vi "Task Killer (pid).vi"(4 "Error In":errorcluster, 6 "Force Kill?":bool, 7 "PID":i32) -> (0 "Error Out":errorcluster)   [LabVIEW 2014, in "Managing Executables.lvlib"]
uses:
  Managing Executables.lvlib
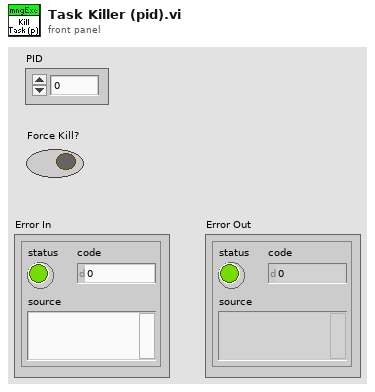
[diagram p1: front panel]
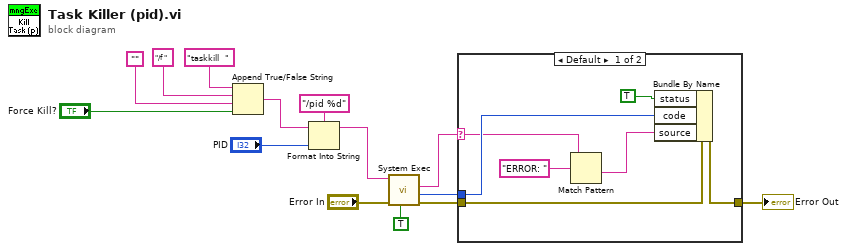
[diagram p0: block diagram]
diagram:
  n1 = Append True/False String(1:"Force Kill?", 2:"" ("format string"), 3:"/f " ("format string"), 4:"taskkill  " ("format string")) -> (0:w1:string)
  n2 = Format Into String(format string="/pid %d", initial string=w1, "PID") -> (resulting string=w2:string)  [unwired: 1 in, 1 out]
  n3 = call <vilib>:"System Exec.vi"("run minimized? (F)"=TRUE, "error in (no error)"="Error In", "command line"=w2) -> ("error out"=w11:errorcluster, "return code"=w10:i32, "standard error"=w12:string)  [unwired: 5 in, 1 out]
  n4 = case shown="Default" w12 {
    selector: w12 -> [w16 _]
    tunnel: [w20 w22] -> w5
    tunnel: w11 -> [w21 w22]
    tunnel: w10 -> [w18 _]
    frame Default {
      n5 = Match Pattern(string=w16, regular expression="ERROR: ") -> (after substring=w15:string)  [unwired: 1 in, 3 out]
      n6 = Bundle By Name(cluster=w21, "status"=TRUE, "code"=w18, "source"=w15) -> (w20:errorcluster)
    }
    frame "" {
    }
  }
  "Error Out" <- w5
